vi "set caption size 2.vi"(8 "error in (no error)":errorcluster, 9 "max caption width":u32=225, 11 "Ctl Refnum in":refnum<vi>) -> (0 "error out":errorcluster, 3 "Ctl Refnum out":refnum<vi>)   [LabVIEW 2015]
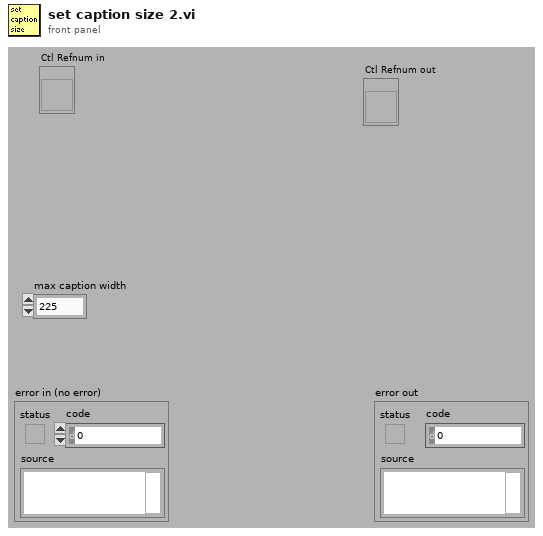
[diagram p1: front panel]
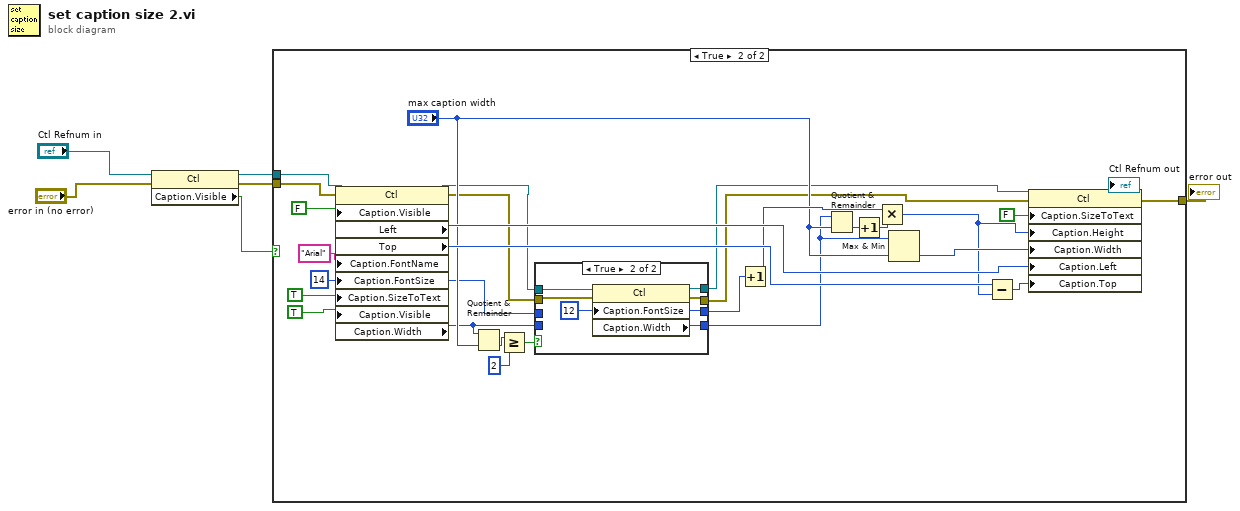
[diagram p0: block diagram]
diagram:
  n1 = property class="Ctl"(reference="Ctl Refnum in", error in="error in (no error)") -> (reference out=w2:refnum<vi>, error out=w3:errorcluster, "Caption.Visible"=w1:bool)
  n2 = case shown="True" w1 {
    tunnel: [w7 w31] -> w6
    tunnel: w3 -> [w7 w29]
    tunnel: w2 -> [_ w28]
    frame False {
    }
    frame True {
      w17 = u32 14 ("Caption.Font:Size")
      n3 = property class="Ctl"(reference=w28, error in=w29, "Caption.Visible"=FALSE, "Caption.FontName"="Arial" ("Caption.Font:Name"), "Caption.FontSize"=w17, "Caption.SizeToText"=TRUE ("Caption.Size to Text?"), "Caption.Visible"=TRUE) -> (reference out=w11:refnum<vi>, error out=w13:errorcluster, "Left"=w25:i32, "Top"=w24:i32, "Caption.Width"=w14:u32)
      n4 = Quotient & Remainder(x=w14, y="max caption width") -> (floor(x/y)=w20:u32)  [unwired: 1 out]
      n5 = Greater Or Equal?(x=w20, y=u32 2) -> (x >= y?=w18:bool)
      n6 = case shown="True" w18 {
        tunnel: w17 -> [w40 _]
        tunnel: [w40 w46] -> w16
        tunnel: [w39 w45] -> w15
        tunnel: w14 -> [w39 _]
        tunnel: w13 -> [w37 w43]
        tunnel: [w37 w44] -> w12
        tunnel: w11 -> [w38 w42]
        tunnel: [w38 w41] -> w10
        frame False {
        }
        frame True {
          w46 = u32 12 ("Caption.Font:Size")
          n7 = property class="Ctl"(reference=w42, error in=w43, "Caption.FontSize"=w46) -> (reference out=w41:refnum<vi>, error out=w44:errorcluster, "Caption.Width"=w45:u32)
        }
      }
      n8 = Increment(x=w16) -> (x+1=w22:u32)
      n9 = Quotient & Remainder(x=w15, y="max caption width") -> (floor(x/y)=w34:u32)  [unwired: 1 out]
      n10 = Increment(x=w34) -> (x+1=w33:u32)
      n11 = Multiply(x=w22, y=w33) -> (x*y=w9:u32)
      n12 = Max & Min(x=w15, y="max caption width") -> (min(x,y)=w30:u32)  [unwired: 1 out]
      n13 = Subtract(x=w24, y=w9) -> (x-y=w35:u32)
      n14 = property class="Ctl"(reference=w10, error in=w12, "Caption.SizeToText"=FALSE ("Caption.Visible"), "Caption.Height"=w9, "Caption.Width"=w30, "Caption.Left"=w25, "Caption.Top"=w35) -> (reference out=→"Ctl Refnum out":refnum<vi>, error out=w31:errorcluster)
    }
  }
  "error out" <- w6
